vi "Untitled 2.vi"() -> ()   [LabVIEW 2014]
uses:
  <vilib>/Instr/_visa.llb/VISA Configure Serial Port (Instr).vi
panel:
  in  "Calibration":bool
  out "Path #3":bool
  out "Path #2":bool
  out "Path #1":bool
  in  "VISA resource name":refnum<visa-resource-name>
  in  "error in (no error)":errorcluster
  out "error out":errorcluster
  out "path detector :":string
  in  "stop":bool
  in  "timeout (100 ms)":u32=10000
  in  "baud rate (115200)":u32=9600
  in  "data bits (8)":u16=8 min=5 max=8 step=1
  in  "parity (0:none)":enum16{"None", "Odd", "Even", "Mark", "Space"}(ring)
  in  "flow control (0:none)":u16(ring) items=["None", "XON/XOFF", "RTS/CTS", "XON/XOFF & RTS/CTS", "DTR/DSR", "XON/XOFF & DTR/DSR"]
  in  "stop bits (10: 1 bit)":u16(ring)=10 items=["1.0"=10, "1.5"=15, "2.0"=20]
  # "NODE 1"
  # "NODE 2"
  # "NODE 3"
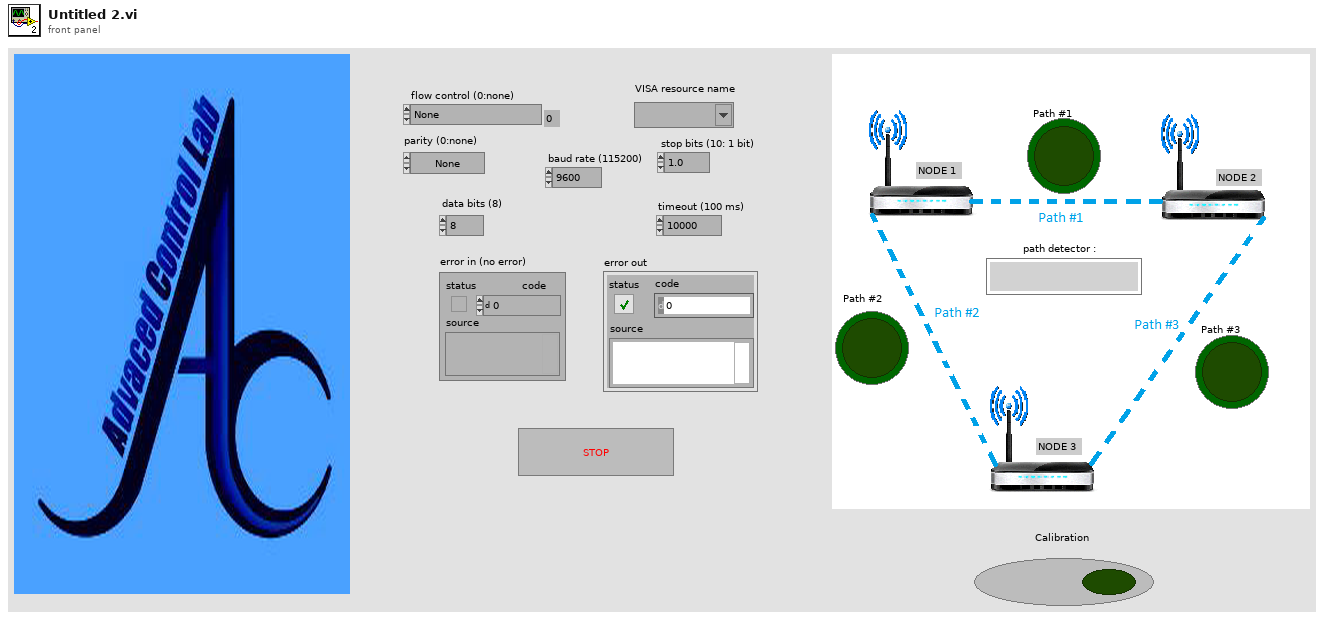
[diagram p1: front panel]
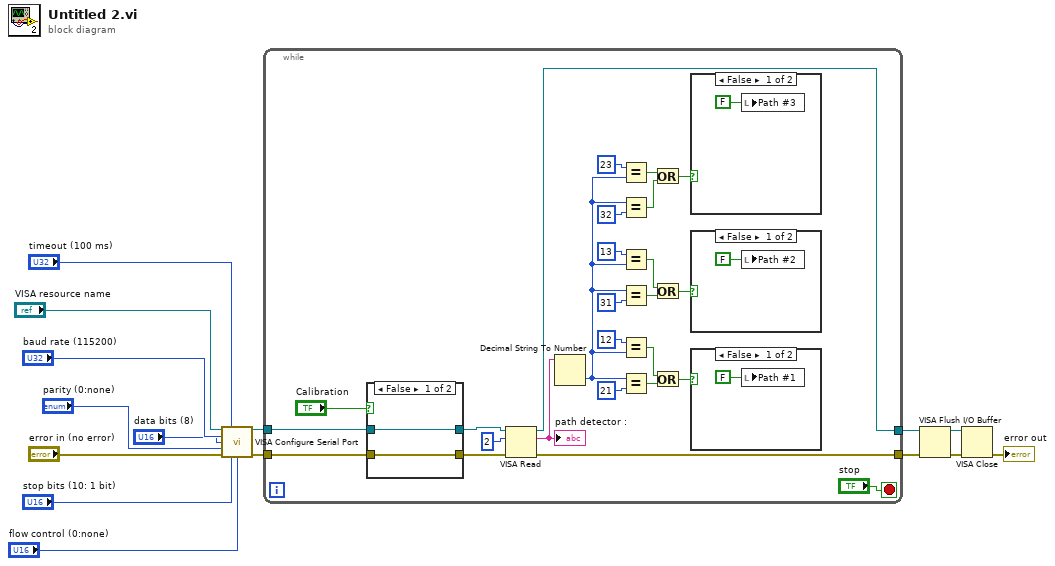
[diagram p0: block diagram]
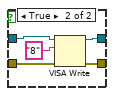
[diagram p2: hidden frame]
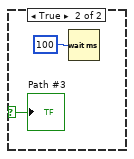
[diagram p3: hidden frame]
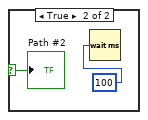
[diagram p4: hidden frame]
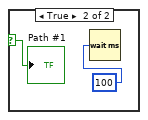
[diagram p5: hidden frame]
diagram:
  n1 = call-poly "VISA Configure Serial Port"("VISA resource name"="VISA resource name", "timeout (10sec)"="timeout (100 ms)", "baud rate (9600)"="baud rate (115200)", "data bits (8)"="data bits (8)", "parity (0:none)"="parity (0:none)", "error in (no error)"="error in (no error)", "stop bits (10: 1 bit)"="stop bits (10: 1 bit)", "flow control (0:none)"="flow control (0:none)") -> ("VISA resource name out"=w7:refnum<visa-resource-name>, "error out"=w8:errorcluster)  [unwired: 6 in]
  n2 = while {
    tunnel: w7 -> [w18]
    tunnel: w8 -> [w19]
    tunnel: [w39] -> w14
    tunnel: [w40] -> w12
    stop <- "stop" stop-if-true
    n3 = case shown="False" "Calibration" {
      tunnel: w19 -> [w43 w48]
      tunnel: [w43 w47] -> w16
      tunnel: [w42 w46] -> w17
      tunnel: w18 -> [w42 w44]
      frame False {
      }
      frame True {
        n4 = VISA Write(VISA resource name=w44, write buffer="8", error in (no error)=w48) -> (VISA resource name out=w46:refnum<visa-resource-name>, error out=w47:errorcluster)  [unwired: 1 out]
      }
    }
    n5 = VISA Read(VISA resource name=w17, byte count=2, error in (no error)=w16) -> (VISA resource name out=w40:refnum<visa-resource-name>, read buffer=w21:string, error out=w39:errorcluster)  [unwired: 1 out]
    "path detector :" <- w21
    n6 = Decimal String To Number(string=w21) -> (number=w35:i32)  [unwired: 2 in, 1 out]
    n7 = Equal?(x=23, y=w35) -> (x = y?=w23:bool)
    n8 = Equal?(x=w35, y=32) -> (x = y?=w24:bool)
    n9 = Equal?(x=13, y=w35) -> (x = y?=w28:bool)
    n10 = Equal?(x=w35, y=31) -> (x = y?=w30:bool)
    n11 = Equal?(x=12, y=w35) -> (x = y?=w33:bool)
    n12 = Equal?(x=w35, y=21) -> (x = y?=w31:bool)
    n13 = Or(x=w23, y=w24) -> (x .or. y?=w25:bool)
    n14 = Or(x=w28, y=w30) -> (x .or. y?=w36:bool)
    n15 = Or(x=w33, y=w31) -> (x .or. y?=w37:bool)
    n16 = case shown="False" w25 {
      selector: w25 -> [_ w51]
      frame False {
        n17 = local write "Path #3"(FALSE ("node #3")) -> ()
      }
      frame True {
        n18 = Wait (ms)(milliseconds to wait=u32 100) -> ()  [unwired: 1 out]
        "Path #3" <- w51
      }
    }
    n19 = case shown="False" w36 {
      selector: w36 -> [_ w54]
      frame False {
        n20 = local write "Path #2"(FALSE ("node #2")) -> ()
      }
      frame True {
        n21 = Wait (ms)(milliseconds to wait=u32 100 ("millisecond timer value")) -> ()  [unwired: 1 out]
        "Path #2" <- w54
      }
    }
    n22 = case shown="False" w37 {
      selector: w37 -> [_ w57]
      frame False {
        n23 = local write "Path #1"(FALSE ("node #1")) -> ()
      }
      frame True {
        n24 = Wait (ms)(milliseconds to wait=u32 100 ("millisecond timer value")) -> ()  [unwired: 1 out]
        "Path #1" <- w57
      }
    }
  }
  n25 = VISA Flush I/O Buffer(VISA resource name=w12, error in (no error)=w14) -> (VISA resource name out=w13:refnum<visa-resource-name>, error out=w15:errorcluster)  [unwired: 1 in]
  n26 = VISA Close(VISA resource name=w13, error in (no error)=w15) -> (error out=→"error out":errorcluster)
